vi "Done.vi"(8 "error in (no error)":errorcluster, 11 "Buffered Log Sink in":refnum<class "Buffered String Log Sink.lvclass">) -> (0 "error out":errorcluster)   [LabVIEW 2019, in "Buffered String Log Sink.lvclass"]
doc: "--\nCopyright © 2017 Composed SystemsI All rights reserved.\n\nAuthor: Jon McBee <jon.mcbee@composed.io>\n\nThis library is provided \"AS IS\" ,WITHOUT WARRANTIES OR\nCONDITIONS OF ANY KIND, either express or implied.\n\nComposed Systems -- composed.io\n\nStream 0.0.1.1\nJon McBee - Composed Systems\nCopyright (c) 2017, Composed Systems"
uses:
  Buffered String Log Sink.lvclass
  Buffered String Log Sink.lvclass/Buffered String Log Sink.ctl
  Composed Log/Log Sink/Log Sink.lvclass
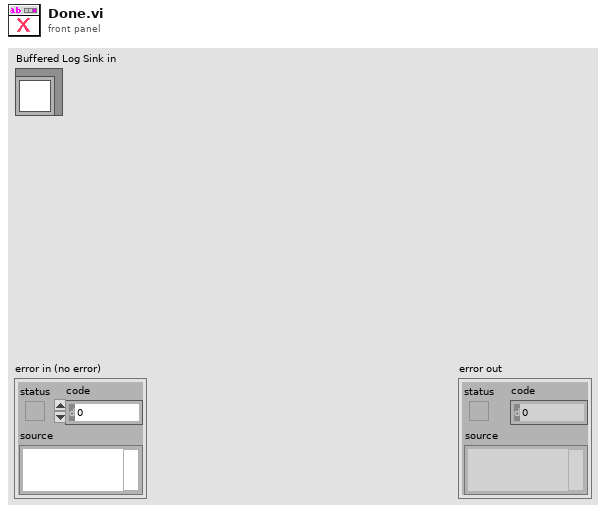
[diagram p1: front panel]
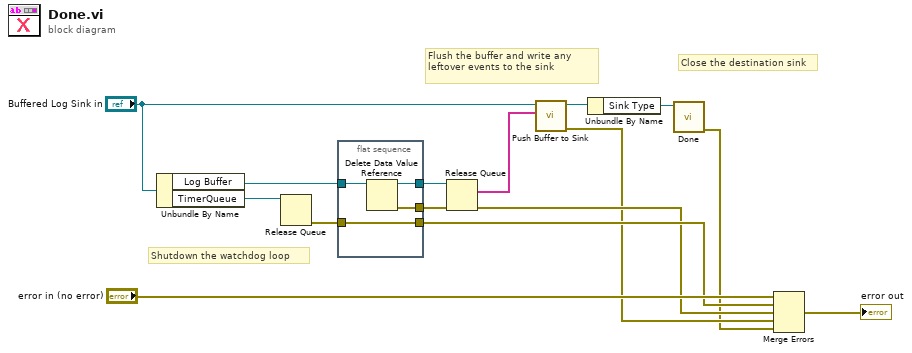
[diagram p0: block diagram]
diagram:
  # "Close the destination sink"
  # "Flush the buffer and write any leftover events to the sink"
  # "Shutdown the watchdog loop"
  n1 = Unbundle By Name("Buffered Log Sink in") -> ("Log Buffer"=w14:refnum<data-value>, "TimerQueue"=w15:refnum<queue>)
  n2 = Release Queue(queue=w15) -> (error out=w13:errorcluster)  [unwired: 2 in, 2 out]
  n3 = flat-sequence {
    tunnel: w14 -> [w19]
    tunnel: w13 -> [w17]
    tunnel: [w18] -> w12
    tunnel: [w17] -> w6
    tunnel: [w16] -> w8
    frame #0 {
      n4 = Delete Data Value Reference(data value reference=w19) -> (data value=w18:refnum<queue>, error out=w16:errorcluster)  [unwired: 1 in]
    }
  }
  n5 = Release Queue(queue=w12, error in (no error)=w8) -> (remaining elements=w10:string[], error out=w5:errorcluster)  [unwired: 1 in, 1 out]
  n6 = call "Push Buffer to Sink.vi"("Strings to Log"=w10, "Buffered Log Sink in"="Buffered Log Sink in") -> ("error out"=w4:errorcluster, "Buffered Log Sink out"=w9:refnum<class "Buffered String Log Sink.lvclass">)  [unwired: 8 in]
  n7 = Unbundle By Name(w9) -> ("Sink Type"=w1:refnum<class "Log Sink.lvclass">)
  n8 = call-dynamic "Done.vi"("Log Sink in"=w1) -> ("error out"=w2:errorcluster)  [unwired: 10 in]
  n9 = Merge Errors("error in (no error)", w6, w5, w4, w2) -> (→"error out":errorcluster)
